vi "Dynamic Load Pulse Drivers.vi"(8 "Error In":errorcluster) -> (0 "Error Out":errorcluster, 2 "Device names":string[](array[string]), 3 "Drivers out":refnum<class "Pulse Driver.lvclass">[](array[class]))   [LabVIEW 2016]
uses:
  Pulse Driver/Pulse Driver.lvclass
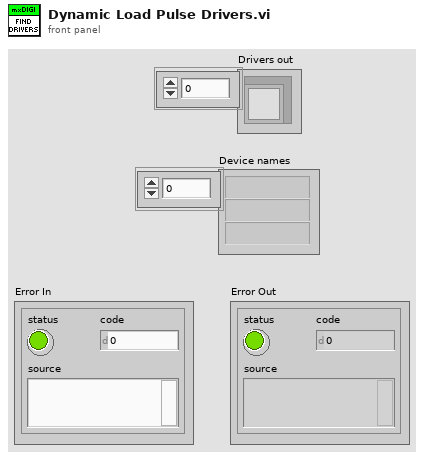
[diagram p1: front panel]
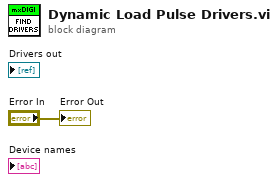
[diagram p0: block diagram]
diagram:
  "Error Out" <- "Error In"
